vi "PH_GetCountRates.vi"() -> ()   [LabVIEW 2019]
panel:
  out "Waveform Graph":dbl[][](graph)
  out "Array2D/SyncRateCH1Rate":dbl[][](array[numeric])
  in  "stop":bool
  in  "PH_Settings_Params":T1={"SyncDiv"=1, "DeviceIndex"=0, "CFD0 level"=50, "CFD0 zero X"=10, "CFD1 level"=50, "CFD1 zero X"=10, "Range No."=0, "StopOnOverflow"=FALSE, "AcqTime (ms)"=0.0} {"Range No." min=0 max=5 step=1; "CFD1 zero X" min=0 max=40 step=1; "CFD1 level" min=0 max=400 step=1; "CFD0 zero X" min=-1300 max=400 step=10; "CFD0 level" min=-1300 max=400 step=10; "SyncDiv" min=1 max=8 step=1}
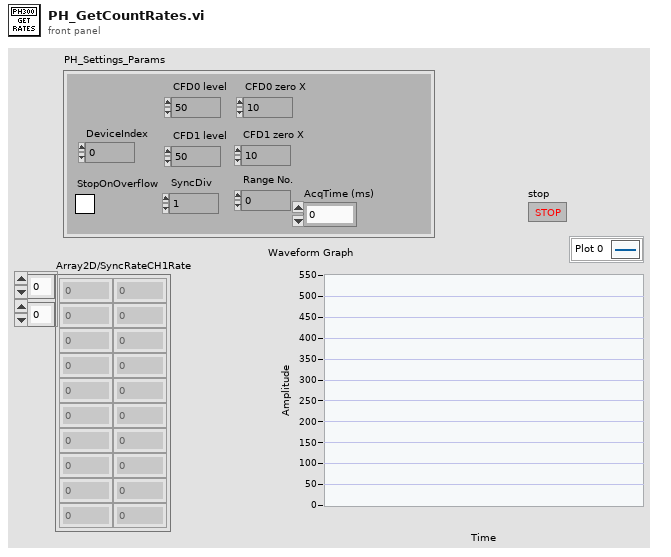
[diagram p1: front panel]
types:
  T1 = cluster{"SyncDiv":i32, "DeviceIndex":i32, "CFD0 level":i32, "CFD0 zero X":i32, "CFD1 level":i32, "CFD1 zero X":i32, "Range No.":i32, "StopOnOverflow":bool, "AcqTime (ms)":dbl}
  T2 = cluster{"Deviceindex":i32, "Initialization Status":string, "DLL Version":string, "Initialization Error":bool, "Status":string, "Calib Error":bool}
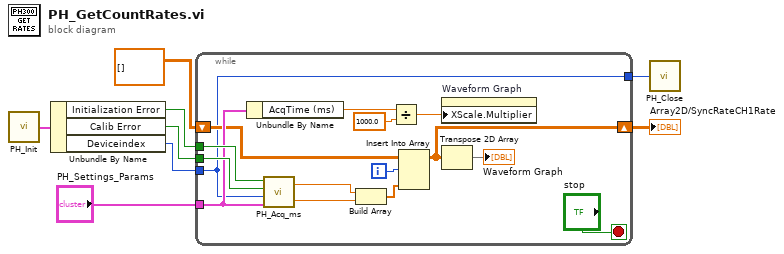
[diagram p0: block diagram]
diagram:
  n1 = call "PH_Init.vi"() -> ("PH_Init_Data"=w8:T2)
  n2 = Unbundle By Name(w8) -> ("Initialization Error"=w7:bool, "Calib Error"=w6:bool, "Deviceindex"=w5:i32)
  n3 = while {
    tunnel: w7 -> [w23]
    tunnel: w6 -> [w22]
    tunnel: w5 -> [w14]
    tunnel: "PH_Settings_Params" -> [w20]
    tunnel: [w14] -> w1
    shift-right: [w12] -> w2
    shift-left: dbl[][] [] -> [w19]
    i -> [w16]
    stop <- "stop" stop-if-true
    n4 = Unbundle By Name(w20) -> ("AcqTime (ms)"=w10:dbl)
    n5 = call "PH_Acq_ms.vi"("PH_Settings_Params"=w20, "Deviceindex"=w14, "Calib Error"=w22, "Initialization Error"=w23) -> ("CH1MeanRate"=w17:dbl, "SyncMeanRate"=w18:dbl)
    n6 = Build Array(w18, w17) -> (w13:dbl[])
    n7 = Divide(x=w10, y=1000.0) -> (x/y=w9:dbl)
    n8 = Insert Into Array(array=w19, index (row)=w16, new element=w13) -> (w12:dbl[][])  [unwired: 1 in]
    n9 = property on="Waveform Graph" class="WFGraph (strict)"("XScale.Multiplier"=w9) -> ()  [unwired: 2 in, 2 out]
    n10 = Transpose 2D Array(2D array=w12) -> (transposed array=→"Waveform Graph":dbl[][])
  }
  "Array2D/SyncRateCH1Rate" <- w2
  n11 = call "PH_Close.vi"("devidx"=w1) -> ()
